vi "Giro_Motor.vi"() -> ()   [LabVIEW 2017]
uses:
  <vilib>/picture/3D Picture Control/NI_3D Picture Control.lvlib
panel:
  in  "Stop Button":bool
  in  "Angulo":dbl(knob) scale=0.0..360.0
  out "Archivos":i32
  out "3D Picture":refnum<vi>(3d-picture)
  in  "Objetos":path=path "C:/Users/LuisFernando/Documents/UPIITA/8vo semestre/Instrumentacion Virtual Aplicada/Modelo_Motor"
  in  "Mundo":path=path "C:/Users/LuisFernando/Documents/UPIITA/8vo semestre/Instrumentacion Virtual Aplicada/Modelo_Motor/Mundo/integracion.wrl"
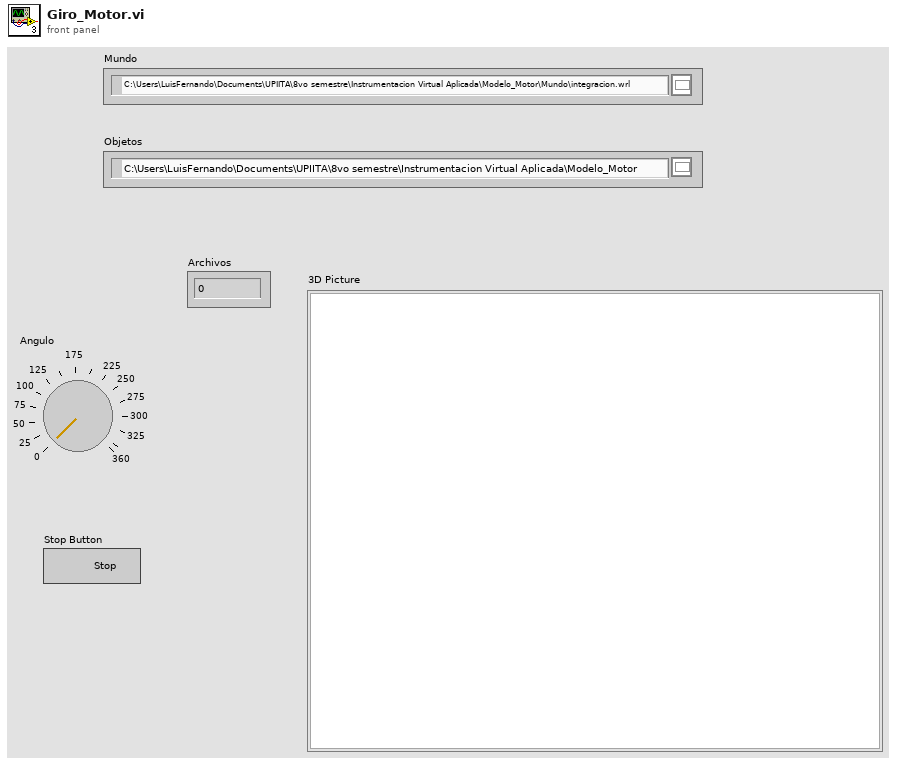
[diagram p1: front panel]
types:
  T1 = enum16{"open", "replace", "create", "open or create", "replace or create", "replace or create with confirmation"}
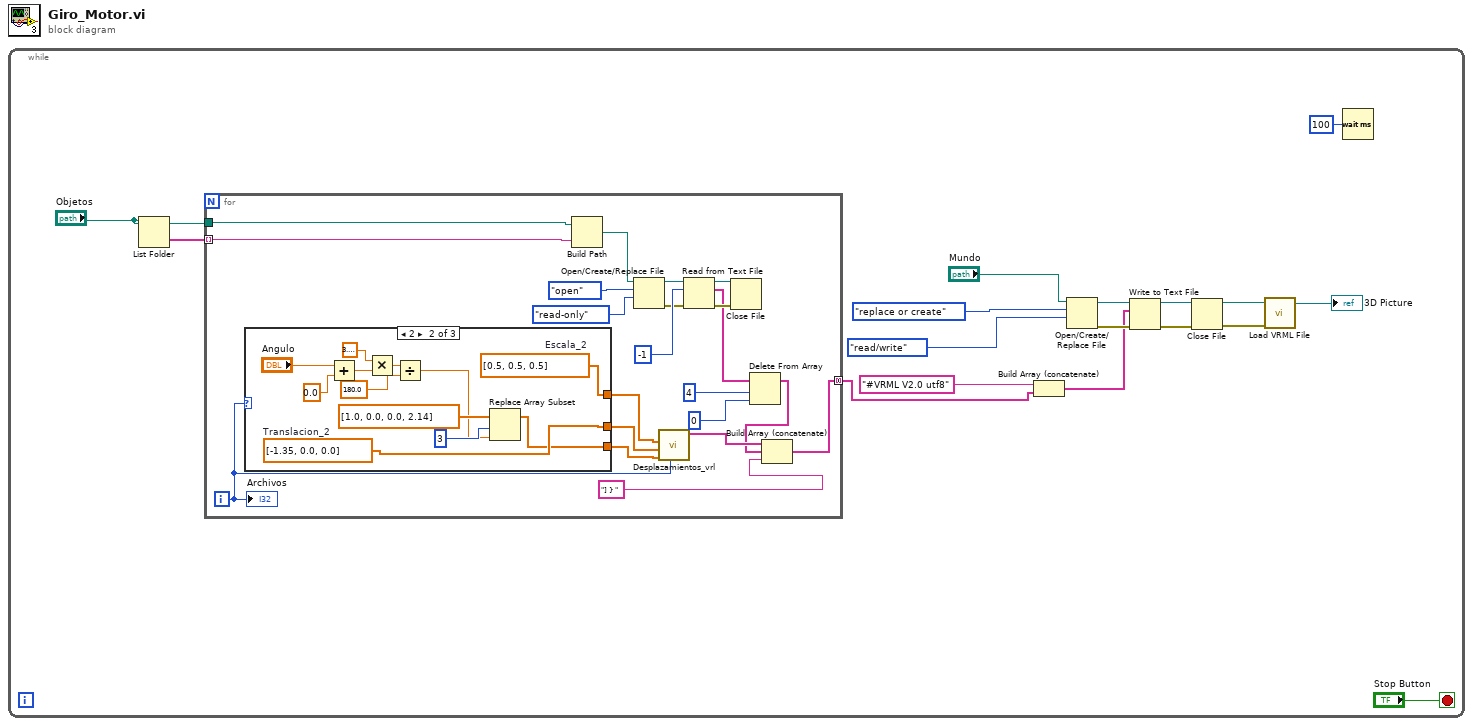
[diagram p0: block diagram]
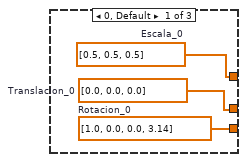
[diagram p2: hidden frame]
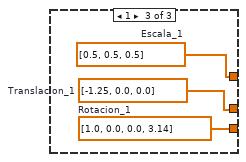
[diagram p3: hidden frame]
diagram:
  n1 = while {
    stop <- "Stop Button" stop-if-true
    n2 = List Folder(path="Objetos") -> (filenames=w10:string[])  [unwired: 3 in, 3 out]
    n3 = for {
      tunnel: w10 -> [w38] mode=indexing
      tunnel: "Objetos" -> [w37]
      tunnel: [w25] -> w5 mode=concatenating
      i -> [w21]
      n4 = case shown="2" w21 {
        tunnel: [w41 w43 w56] -> w20
        tunnel: [w40 w44 w55] -> w19
        tunnel: [w39 w45 w54] -> w18
        frame 0, Default {
          w41 = dbl[] [1.0, 0.0, 0.0, 3.14]  # Rotacion_0
          w40 = dbl[] [0.0, 0.0, 0.0]  # Translacion_0
          w39 = dbl[] [0.5, 0.5, 0.5]  # Escala_0
        }
        frame 2 {
          w44 = dbl[] [-1.35, 0.0, 0.0]  # Translacion_2
          w45 = dbl[] [0.5, 0.5, 0.5]  # Escala_2
          n5 = Add(x="Angulo", y=0.0) -> (x+y=w53:dbl)
          n6 = Multiply(x=3.141592653589793, y=w53) -> (x*y=w52:dbl)
          n7 = Divide(x=w52, y=180.0) -> (x/y=w42:dbl)
          n8 = Replace Array Subset(array=dbl[] [1.0, 0.0, 0.0, 2.14] ("Rotacion_2"), new element=w42, index=3) -> (w43:dbl[])
        }
        frame 1 {
          w56 = dbl[] [1.0, 0.0, 0.0, 3.14]  # Rotacion_1
          w55 = dbl[] [-1.25, 0.0, 0.0]  # Translacion_1
          w54 = dbl[] [0.5, 0.5, 0.5]  # Escala_1
        }
      }
      n9 = Build Path(base path=w37, name or relative path=w38) -> (appended path=w36:path)
      n10 = Open/Create/Replace File(file path (use dialog)=w36, operation (0:open)=T1."open", access (0:read/write)=enum16{"read/write", "read-only", "write-only"}."read-only") -> (refnum out=w33:refnum<file>, error out=w31:errorcluster)  [unwired: 3 in, 1 out]
      n11 = call "Desplazamientos_vrl.vi"("Indice"=w21, "Rotacion"=w20, "Translacion"=w19, "Escala"=w18) -> ("Salida"=w23:string[])  [unwired: 7 in]
      n12 = Read from Text File(file (use dialog)=w33, count=-1, error in=w31) -> (refnum out=w29:refnum<file>, text=w26:string[], error out=w30:errorcluster)  [unwired: 1 in, 1 out]
      n13 = Close File(refnum=w29, error in=w30) -> ()  [unwired: 2 out]
      n14 = Delete From Array(array=w26, length=4, index=0) -> (array with subset deleted=w22:string[])  [unwired: 1 out]
      n15 = Build Array (concatenate)(w23, w22, "] } ") -> (w25:string[])
      "Archivos" <- w21
    }
    n16 = Build Array (concatenate)("#VRML V2.0 utf8", w5) -> (w4:string[])
    n17 = Open/Create/Replace File(file path (use dialog)="Mundo", operation (0:open)=T1."replace or create", access (0:read/write)=enum16{"read/write", "read-only", "write-only"}."read/write") -> (refnum out=w14:refnum<file>, error out=w13:errorcluster)  [unwired: 3 in, 1 out]
    n18 = Write to Text File(file (use dialog)=w14, text=w4, error in=w13) -> (refnum out=w11:refnum<file>, error out=w12:errorcluster)  [unwired: 1 in, 1 out]
    n19 = Close File(refnum=w11, error in=w12) -> (path=w8:path, error out=w7:errorcluster)
    n20 = call <vilib>:"Load VRML File.vi"("error in"=w7, "Path"=w8) -> ("Scene:Read Scene File"=→"3D Picture":refnum<vi>)  [unwired: 8 in, 1 out]
    n21 = Wait (ms)(milliseconds to wait=u32 100) -> ()  [unwired: 1 out]
  }
